vi "MU Create Mt Sync.vi"(8 "error in (no error)":errorcluster, 9 "mtMovementIsReverse":bool, 10 "nMtSyncBits":u64, 11 "CalibrationHandle":T1) -> (0 "error out":errorcluster, 3 "mtSyncHandle":T2)   [LabVIEW 2017, in "MU_3SL_interface.lvlib"]
uses:
  MU_3SL_interface.lvlib
  handles/mtSyncHandle.ctl
  handles/CalibrationHandle.ctl
  lib/MU_3SL_interface.dll
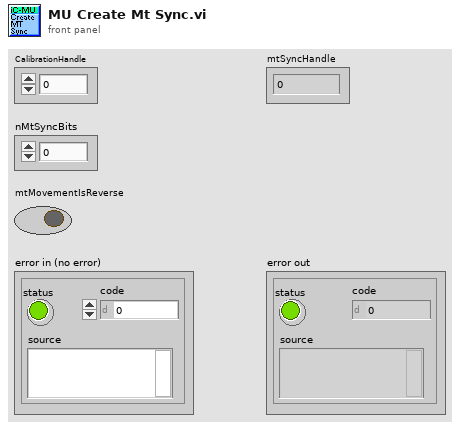
[diagram p1: front panel]
types:
  T1 = typedef "MU_3SL_interface.lvlib/CalibrationHandle.ctl" = u64
  T2 = typedef "MU_3SL_interface.lvlib/mtSyncHandle.ctl" = u64
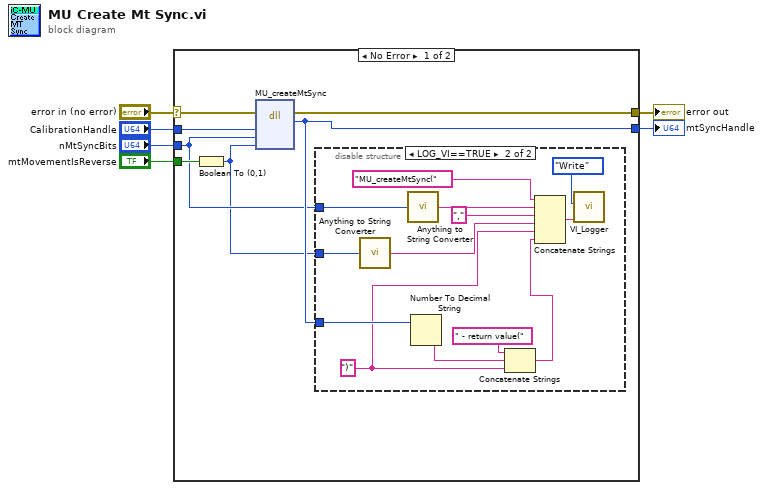
[diagram p0: block diagram]
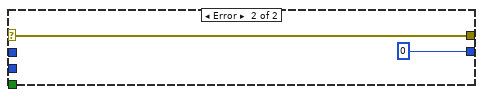
[diagram p3: hidden frame]
diagram:
  n1 = case shown="No Error" "error in (no error)" {
    selector: "error in (no error)" -> [w13 w28]
    tunnel: [w11 u64 0 ("mtSynchHandle")] -> w4
    tunnel: [w10 w28] -> w6
    tunnel: "CalibrationHandle" -> [w12 _]
    tunnel: "nMtSyncBits" -> [w8 _]
    tunnel: "mtMovementIsReverse" -> [w9 _]
    frame No Error {
      n2 = Boolean To (0,1)(Boolean=w9) -> (0, 1=w7:i16)
      n3 = dll-call lib="C:/Users/bes/AppData/Roaming/work/mu_9so/icsubmodules/soft_mu_3sl_master/lv_interface/lib/MU_3SL_interface**.*" fn="MU_createMtSync"(error in=w13, "CalibrationHandle"=w12, "nMtSyncBits"=w8, "mtMovementIsReverse"=w7) -> (error out=w10:errorcluster, "mtSyncHandle"=w11:u64)  [unwired: 5 in, 1 out]
      n4 = disable-structure shown="LOG_VI==TRUE" {
        disable-tunnel: w11 -> [_ w22]
        disable-tunnel: w8 -> [_ w20]
        disable-tunnel: w7 -> [_ w19]
        frame condition #0 {
        }
        frame condition #1 (active) {
          w15 = ")" ("string")
          n5 = call "Anything to String Converter.vi"("anything"=w19) -> ("String"=w16:string)
          n6 = call "Anything to String Converter.vi"("anything"=w20) -> ("String"=w18:string)
          n7 = Number To Decimal String(number=w22) -> (decimal integer string=w21:string)  [unwired: 1 in]
          n8 = Concatenate Strings(" - return value(" ("string"), w21, w15) -> (w14:string)
          n9 = Concatenate Strings("MU_createMtSync(" ("Info in"), w18, "," ("string"), w16, w15, w14) -> (w24:string)
          n10 = call "VI_Logger.vi"("Action (Read)"=enum16{"Write", "Read"}."Write", "Info in"=w24) -> ()  [unwired: 8 in, 2 out]
        }
      }
    }
    frame Error {
    }
  }
  "error out" <- w6
  "mtSyncHandle" <- w4
